vi "ReadPowerSupplies.vi"(11 "error in (no error)":errorcluster) -> (2 "Idd":string, 3 "IddA":string, 4 "IddNB":string, 6 "IddIO":string, 8 "Itt":string, 10 "Ildt":string, 15 "error out":errorcluster)   [LabVIEW 2011]
doc: "This VI reads all of the power supplies current draw.\n\nOutputs:\n1. Idd/IddA/IddNB/IddIO/Itt/Ildt: The current draw read from each power supply."
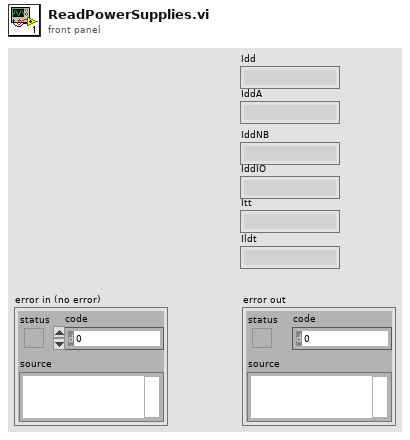
[diagram p1: front panel]
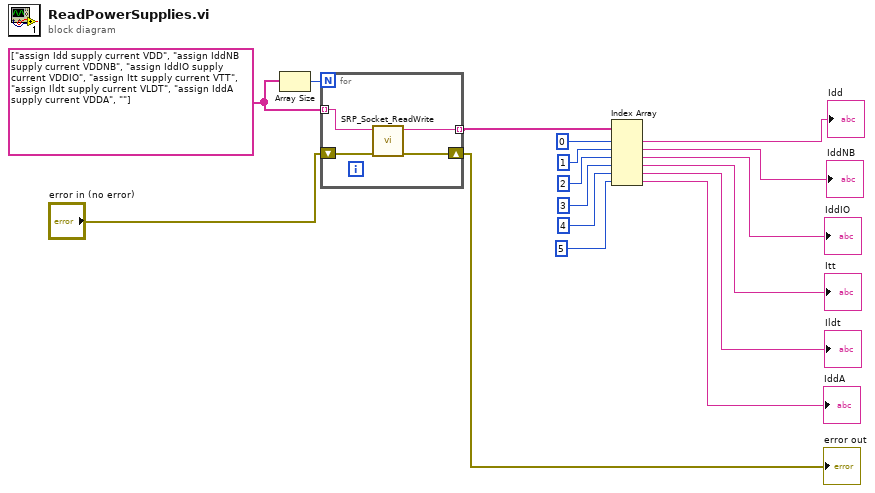
[diagram p0: block diagram]
diagram:
  w16 = string[] ["assign Idd supply current VDD", "assign IddNB supply current VDDNB", "assign IddIO supply current VDDIO", "assign Itt supply current VTT", "assign Ildt supply current VLDT", "assign IddA supply current VDDA", ""]
  n1 = Array Size(array=w16) -> (size(s)=w17:i32)
  n2 = for {
    N: w17 -> [_]
    tunnel: w16 -> [w19] mode=indexing
    shift-right: [w21] -> w14
    shift-left: "error in (no error)" -> [w20]
    tunnel: [w18] -> w1 mode=indexing
    n3 = call "SRP_Socket_ReadWrite.vi"("error in (no error)"=w20, "Data In"=w19) -> ("error out"=w21:errorcluster, "Data Out"=w18:string)  [unwired: 7 in]
  }
  "error out" <- w14
  n4 = Index Array(array=w1, index #1=0 ("index"), index #2=1 ("index"), index #3=2 ("index"), index #4=3 ("index"), index #5=4 ("index"), index #6=5 ("index")) -> (element #1=→"Idd":string, element #2=→"IddNB":string, element #3=→"IddIO":string, element #4=→"Itt":string, element #5=→"Ildt":string, element #6=→"IddA":string)
